vi "niRFUtil MASMT Resample (constant to constant)_Resample (DBL).vi"(4 "max decimation":i32=1000, 6 "Resample FIR":dbl[](array[numeric]), 7 "reset?":bool, 8 "error in (no error)":errorcluster, 9 "config":T1 {"timing jitter" items=["Interpolation", "Rounding"]}, 10 "anti-aliasing?":bool=TRUE, 11 "X":dbl[](array[numeric])) -> (0 "error out":errorcluster, 2 "t0":dbl, 3 "Y":dbl[](array[numeric]))   [LabVIEW 2015, in "niRFUtil.lvlib"]
uses:
  niRFUtil.lvlib
  Utilities/niRFMASMT_FFT.dll
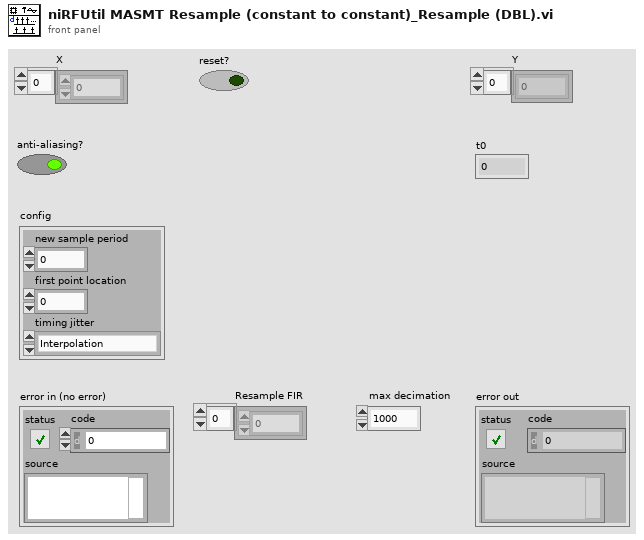
[diagram p1: front panel]
types:
  T1 = cluster{"new sample period":dbl, "first point location":dbl, "timing jitter":i32}
  T2 = cluster{"preConditionLen":i32, "extractFilterLeftLen":i32, "extractFilterRightLen":i32, "extractFilterMethod":i32, "extractFilterScaling":dbl, "samplingPeriod":dbl, "startTime":dbl, "offset":dbl, "index":i32}
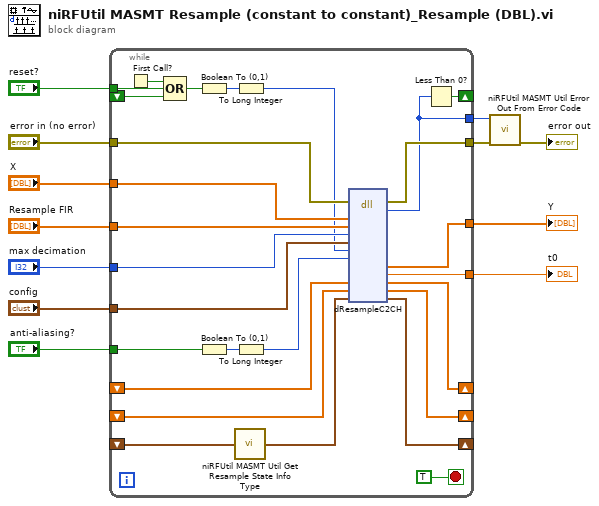
[diagram p0: block diagram]
diagram:
  n1 = while {
    tunnel: "X" -> [w39]
    tunnel: "config" -> [w38]
    tunnel: "error in (no error)" -> [w37]
    tunnel: [w36] -> w5
    tunnel: "anti-aliasing?" -> [w35]
    tunnel: "Resample FIR" -> [w33]
    tunnel: "max decimation" -> [w32]
    tunnel: [w20] -> w3
    tunnel: [w30] -> w2
    tunnel: [w29] -> w4
    tunnel: "reset?" -> [w18]
    shift-right: [w26] -> _
    shift-left: _ -> [w23]
    shift-right: [w27] -> _
    shift-left: _ -> [w22]
    shift-right: [w19] -> _
    shift-left: _ -> [w17]
    shift-right: [w25] -> _
    shift-left: _ -> [w13]
    stop <- TRUE stop-if-true
    n2 = First Call?() -> (First Call?: T/F=w14:bool)
    n3 = Compound Arithmetic op=OR(w14, w18, w17) -> (w15:bool)
    n4 = Boolean To (0,1)(Boolean=w15) -> (0, 1=w16:i16)
    n5 = Boolean To (0,1)(Boolean=w35) -> (0, 1=w34:i16)
    n6 = call "niRFUtil MASMT Util Get Resample State Info Type.vi"("resample state info in"=w22) -> ("resample state info out"=w21:T2)
    n7 = To Long Integer(number=w16) -> (32bit integer=w28:i32)
    n8 = To Long Integer(number=w34) -> (32bit integer=w31:i32)
    n9 = dll-call lib="C:/Perforce/semoore-sales/Customers/NATI-3813/Noise Floor/LV Filters/ParallelComplexFilterRFUtil/niRFUtil/MASMT/Utilities/niRFMASMT_FFT.*" fn="dResampleC2CH"(error in=w37, "xH"=w39, "pfilterCoefH"=w33, "pfilterMaxDecimation"=w32, "config"=w38, "reset"=w28, "bandLimit"=w31, "xBufferH"=w23, "extractFilterH"=w13, "state"=w21) -> (error out=w30:errorcluster, "error"=w20:i32, "yH"=w29:dbl[], "t0"=w36:dbl, "xBufferH"=w26:dbl[], "extractFilterH"=w25:dbl[], "state"=w27:T2)  [unwired: 10 in, 1 out]
    n10 = Less Than 0?(x=w20) -> (x < 0?=w19:bool)
  }
  "t0" <- w5
  "Y" <- w4
  n11 = call "niRFUtil MASMT Util Error Out From Error Code.vi"("error in (no error)"=w2, "error code"=w3) -> ("error out"=→"error out":errorcluster)  [unwired: 9 in]
